vi "baratron_conversion_CDG1.vi"(10 "V_CDG1 (V)":dbl) -> (2 "y (Pa)":dbl)   [LabVIEW 2017]
uses:
  <vilib>/express/express arith-compare/Formula/XNode/ExpressFormulaBlockNode.xnode
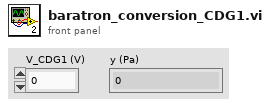
[diagram p1: front panel]
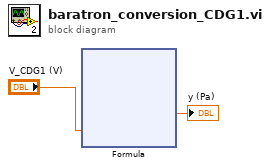
[diagram p0: block diagram]
diagram:
  n1 = xnode "Formula"("X"="V_CDG1 (V)") -> ("結果"=→"y (Pa)":dbl)  [unwired: 1 in, 1 out]
